vi "BUSDataGenerator.vi"(9 "TestLoops":i32, 10 "dt":dbl, 11 "BUSChannelStructArray":T1) -> (2 "BUSDataArray":u16[](array[numeric]))   [LabVIEW 2011]
uses:
  N:/Ins18Programm/LVRealTimeCore/BUSChannelStructArray.ctl
  N:/Ins18Programm/LVRealTimeCore/BUSChannelStruct.ctl
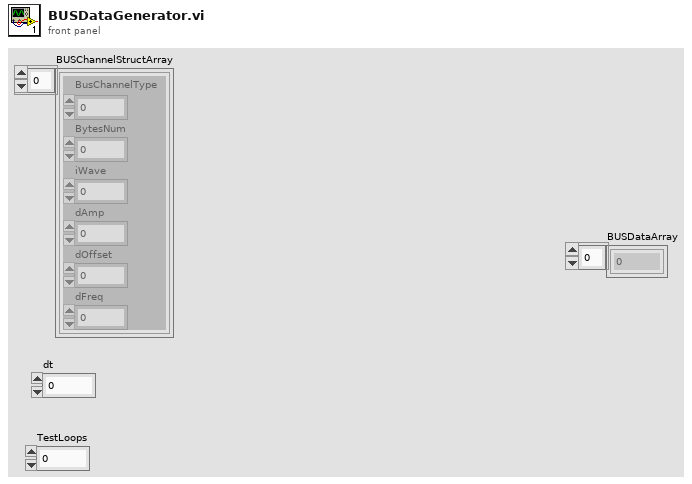
[diagram p1: front panel]
types:
  T1 = typedef "BUSChannelStructArray.ctl" = T2[]
  T2 = typedef "BUSChannelStruct.ctl" = cluster{"BusChannelType":i32, "BytesNum":i32, "iWave":i32, "dAmp":i16, "dOffset":i16, "dFreq":dbl}
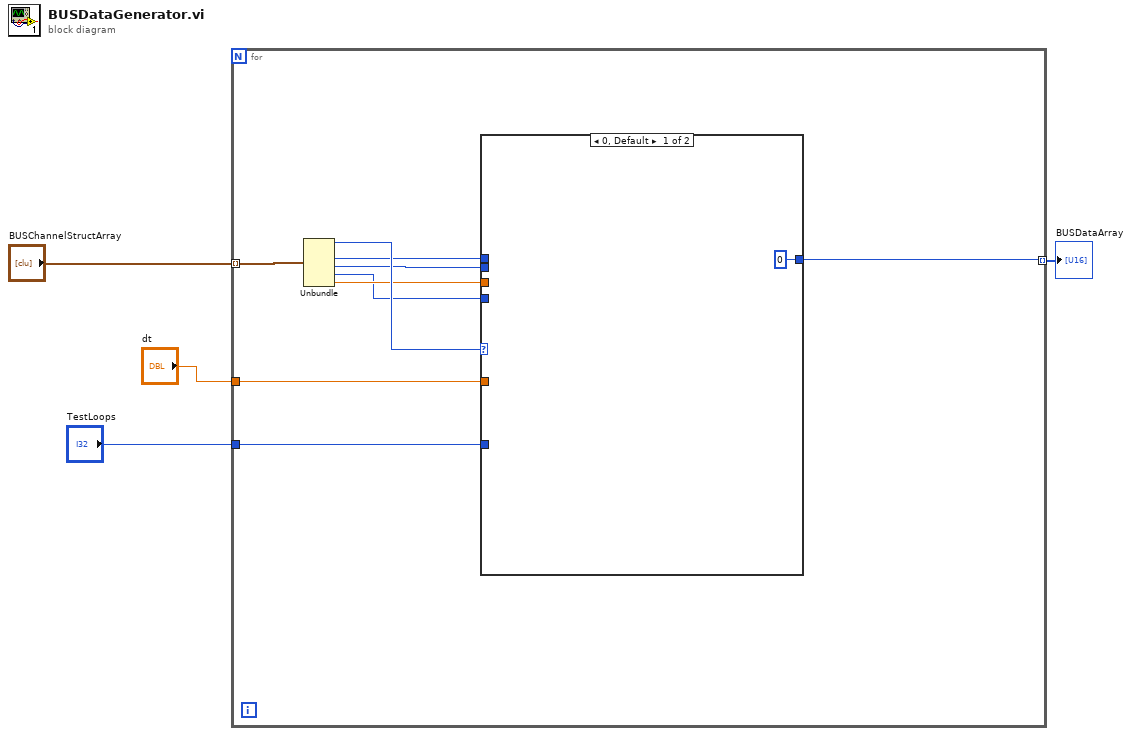
[diagram p0: block diagram]
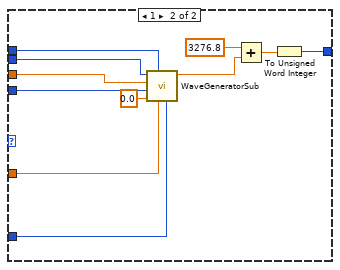
[diagram p2: hidden frame]
diagram:
  n1 = for {
    tunnel: "BUSChannelStructArray" -> [w13] mode=indexing
    tunnel: "dt" -> [w7]
    tunnel: "TestLoops" -> [w6]
    tunnel: [w5] -> w1 mode=indexing
    n2 = Unbundle(w13) -> ("BusChannelType"=w12:i32, "iWave"=w8:i32, "dAmp"=w11:i16, "dOffset"=w9:i16, "dFreq"=w10:dbl)  [unwired: 1 out]
    n3 = case shown="0, Default" w12 {
      tunnel: w11 -> [_ w25]
      tunnel: w10 -> [_ w24]
      tunnel: w9 -> [_ w23]
      tunnel: w8 -> [_ w21]
      tunnel: w7 -> [_ w20]
      tunnel: w6 -> [_ w19]
      tunnel: [u16 0 w15] -> w5
      frame 0, Default {
      }
      frame 1 {
        n4 = call "WaveGeneratorSub.vi"("TestLoops"=w19, "dt"=w20, "Wave"=w21, "deltaF"=0.0, "Offset"=w23, "Frequent"=w24, "Amplitude"=w25) -> ("Output"=w18:dbl)  [unwired: 4 in]
        n5 = Add(x=3276.8, y=w18) -> (x+y=w16:dbl)
        n6 = To Unsigned Word Integer(number=w16) -> (unsigned 16bit integer=w15:u16)
      }
    }
  }
  "BUSDataArray" <- w1
